vi "oa_Buffered Output Waveform Data (N Channels).vi"(0 "scaled signal [EU]":waveform(dbl)[](array[waveform]), 1 "reset? (True)":bool=TRUE, 5 "start":dbl[](array[numeric]), 7 "durations":dbl[](array[numeric]), 9 "# of revolutions":dbl, 11 "error in":errorcluster) -> (4 "scaled signal [EU] out":waveform(dbl)[](array[waveform]), 6 "start points":dbl[](array[numeric]), 8 "durations":dbl[](array[numeric]), 10 "total duration":dbl, 15 "error out":errorcluster)   [LabVIEW 2017]
uses:
  <vilib>/Waveform/WDTOps.llb/WDT Get Waveform Subset DBL.vi
  <vilib>/Waveform/WDTOps.llb/WDT Append Waveforms DBL.vi
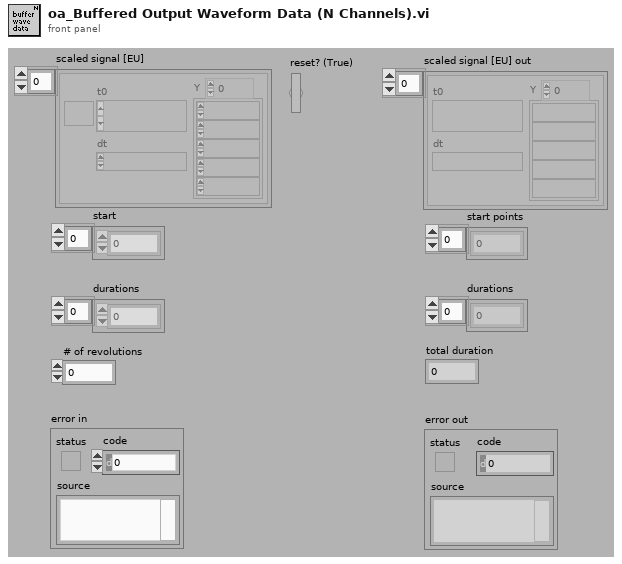
[diagram p1: front panel]
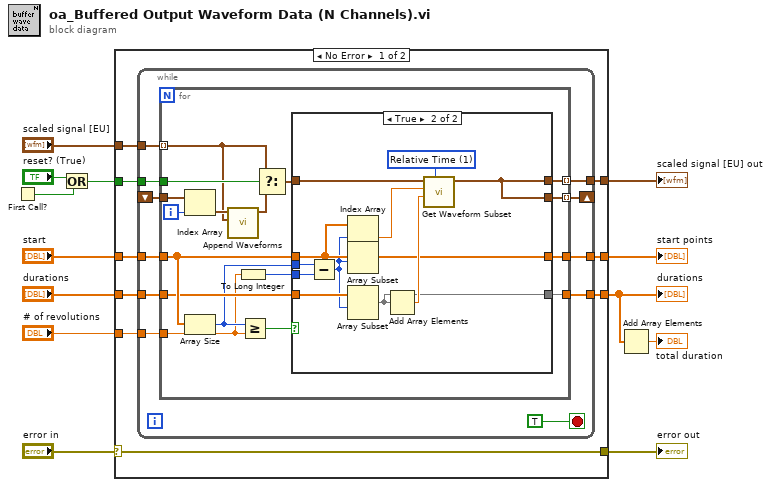
[diagram p0: block diagram]
diagram:
  n1 = First Call?() -> (First Call?: T/F=w2:bool)
  n2 = Or(x="reset? (True)", y=w2) -> (x .or. y?=w1:bool)
  n3 = case shown="No Error" "error in" {
    selector: "error in" -> [w18 w69]
    tunnel: [w18 w69] -> w12
    tunnel: "start" -> [w22 w67]
    tunnel: "# of revolutions" -> [w21 _]
    tunnel: "scaled signal [EU]" -> [w20 w68]
    tunnel: [w19 w68] -> w8
    tunnel: w1 -> [w17 _]
    tunnel: "durations" -> [w16 w66]
    tunnel: [w15 w67] -> w6
    tunnel: [w14 w66] -> w5
    frame No Error {
      n4 = while {
        tunnel: w22 -> [w33]
        tunnel: w21 -> [w32]
        tunnel: w20 -> [w31]
        tunnel: [w30] -> w19
        shift-right: [w28] -> _
        shift-left: _ -> [w27]
        tunnel: w17 -> [w26]
        tunnel: w16 -> [w25]
        tunnel: [w24] -> w15
        tunnel: [w23] -> w14
        stop <- TRUE stop-if-true
        n5 = for {
          tunnel: w33 -> [w40]
          tunnel: w32 -> [w35]
          tunnel: w31 -> [w43] mode=indexing
          tunnel: [w49] -> w30 mode=indexing
          tunnel: [w48] -> w28 mode=indexing
          tunnel: w27 -> [w47]
          tunnel: w26 -> [w44]
          tunnel: w25 -> [w39]
          tunnel: [w38] -> w24
          tunnel: [w37] -> w23
          i -> [w46]
          n6 = Index Array(array=w47, index=w46) -> (element=w45:waveform(dbl))
          n7 = Array Size(array=w40) -> (size(s)=w36:i32)
          n8 = call-poly <vilib>:"Append Waveforms.vi"("waveform B"=w43, "waveform A"=w45) -> ("waveform out"=w42:waveform(dbl))  [unwired: 8 in, 1 out]
          n9 = To Long Integer(number=w35) -> (32bit integer=w34:i32)
          n10 = Greater Or Equal?(x=w36, y=w35) -> (x >= y?=w50:bool)
          n11 = Select(t=w43, s=w44, f=w42) -> (s? t:f=w41:waveform(dbl))
          n12 = case shown="True" w50 {
            tunnel: w41 -> [w53 w62]
            tunnel: [w53 w54] -> w49
            tunnel: [w53 w54] -> w48
            tunnel: w40 -> [w52 w57]
            tunnel: w39 -> [w51 w63]
            tunnel: [w52 w55] -> w38
            tunnel: [w51 w58] -> w37
            tunnel: w36 -> [_ w65]
            tunnel: w34 -> [_ w64]
            frame False {
            }
            frame True {
              w61 = u16 1 items=["Index", "Relative Time"] ("Mode")
              n13 = Subtract(x=w65, y=w64) -> (x-y=w56:i32)
              n14 = Index Array(array=w57, index=w56) -> (element=w60:dbl)
              n15 = Array Subset(array=w57, index=w56) -> (w55:dbl[])  [unwired: 1 in]
              n16 = Array Subset(array=w63, index=w56) -> (w58:dbl[])  [unwired: 1 in]
              n17 = Add Array Elements(numeric array=w58) -> (sum=w59:dbl)
              n18 = call-poly <vilib>:"Get Waveform Subset.vi"("start/duration format"=w61, "duration"=w59, "start samples/time"=w60, "waveform in"=w62) -> ("waveform out"=w54:waveform(dbl))  [unwired: 2 in, 3 out]
            }
          }
        }
      }
    }
    frame Error {
    }
  }
  "error out" <- w12
  "scaled signal [EU] out" <- w8
  "start points" <- w6
  "durations" <- w5
  n19 = Add Array Elements(numeric array=w5) -> (sum=→"total duration":dbl)
